vi "toStringArray.vi"(8 "error in (no error)":errorcluster, 11 "rf in":refnum<class "rf.lvclass">) -> (0 "error out":errorcluster, 2 "eventStringArray":string[](array[string]), 3 "rf out":refnum<class "rf.lvclass">)   [LabVIEW 2011, in "Tools.lvlib" / "Scripting.lvlib" / "rf.lvclass"]
uses:
  rf.lvclass
  ScriptEvent.lvclass
  rf.lvclass/rf.ctl
  DatabaseHelpers/Database Objects/Channel/RfOutputChannel/RfOutputChannel.lvclass
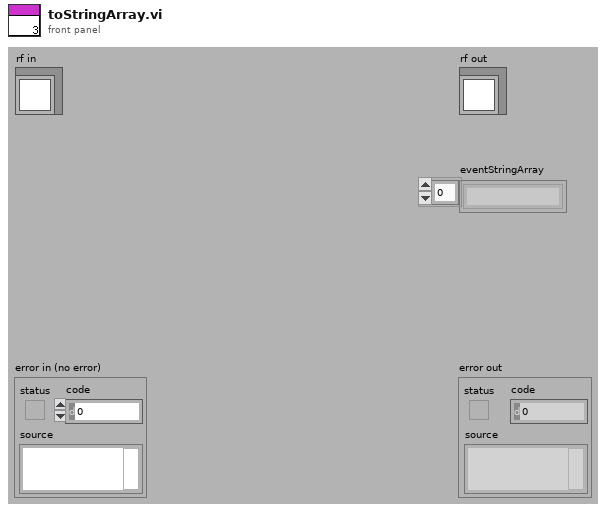
[diagram p1: front panel]
types:
  T1 = cluster{"state_name":string, "value":cluster{"frequency":string, "amplitude":string, "phase":string}}[]
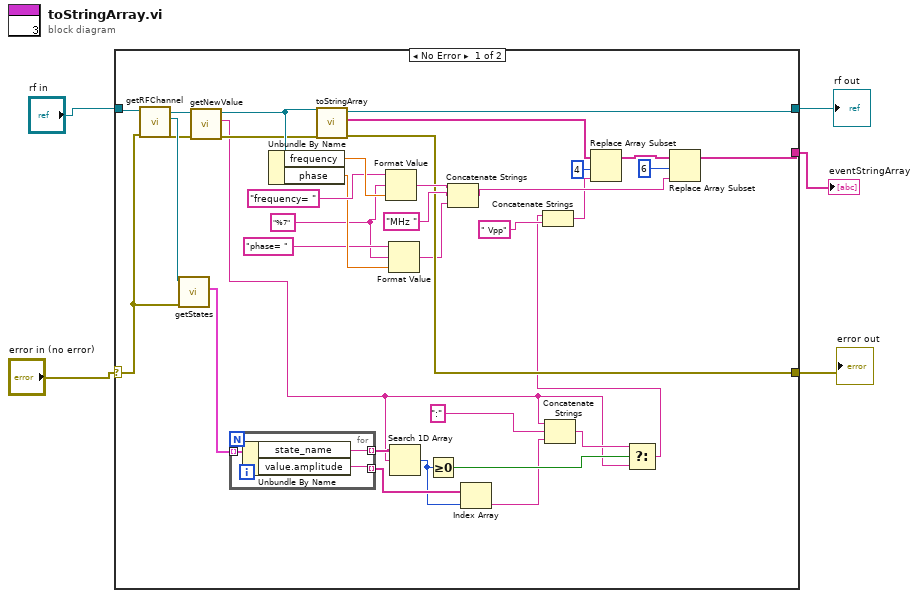
[diagram p0: block diagram]
diagram:
  n1 = case shown="No Error" "error in (no error)" {
    selector: "error in (no error)" -> [w22 w45]
    tunnel: [w32 w45] -> w1
    tunnel: [w40 w44] -> w3
    tunnel: "rf in" -> [w24 w44]
    tunnel: [w33 _] -> w2
    frame No Error {
      w26 = "%7"
      n2 = call "getRFChannel.vi"("error in (no error)"=w22, "rf.lvclass in"=w24) -> ("error out"=w13:errorcluster, "RfOutputChannel.lvclass"=w23:refnum<class "RfOutputChannel.lvclass">, "rf.lvclass out"=w16:refnum<class "rf.lvclass">)  [unwired: 7 in]
      n3 = call "getStates.vi"("error in (no error)"=w22, "RfOutputChannel in"=w23) -> ("states"=w17:T1)  [unwired: 7 in, 2 out]
      n4 = call "getNewValue.vi"("error in (no error)"=w13, "ScriptEvent.lvclass in"=w16) -> ("error out"=w14:errorcluster, "newValue"=w9:string, "ScriptEvent.lvclass out"=w15:refnum<class "rf.lvclass">)  [unwired: 7 in]
      n5 = for {
        tunnel: w17 -> [w43] mode=indexing
        tunnel: [w42] -> w21 mode=indexing
        tunnel: [w41] -> w12 mode=indexing
        n6 = Unbundle By Name(w43) -> ("state_name"=w42:string, "value.amplitude"=w41:string)
      }
      n7 = Unbundle By Name(w15) -> ("frequency"=w38:dbl, "phase"=w28:dbl)
      n8 = call-parent "toStringArray.vi"("error in (no error)"=w14, "ScriptEvent in"=w15) -> ("error out"=w32:errorcluster, "eventStringArray"=w7:string[], "ScriptEvent out"=w40:refnum<class "rf.lvclass">)  [unwired: 7 in]
      n9 = Format Value(string ("")="frequency= ", format string=w26, value (0)=w38) -> (output string=w36:string)
      n10 = Format Value(string ("")="phase= ", format string=w26, value (0)=w28) -> (output string=w25:string)
      n11 = Search 1D Array(1D array=w21, element=w9) -> (index of element=w11:i32)  [unwired: 1 in]
      n12 = Greater Or Equal To 0?(x=w11) -> (x >= 0?=w18:bool)
      n13 = Concatenate Strings(w36, "MHz ", w25) -> (w34:string)
      n14 = Index Array(array=w12, index=w11) -> (element=w10:string)
      n15 = Concatenate Strings(w9, ":", w10) -> (w19:string)
      n16 = Select(t=w19, s=w18, f=w9) -> (s? t:f=w8:string)
      n17 = Concatenate Strings(w8, " Vpp") -> (w29:string)
      n18 = Replace Array Subset(array=w7, new element=w29, index=4) -> (w6:string[])
      n19 = Replace Array Subset(array=w6, new element=w34, index=6) -> (w33:string[])
    }
    frame Error {
    }
  }
  "error out" <- w1
  "rf out" <- w3
  "eventStringArray" <- w2
